vi "read.vi"(7 "timeout (ms)":i32, 8 "error in (no error)":errorcluster, 9 "number of channels":i32, 10 "block size":i32, 11 "FPGAWrapperDL090211Galvo in":refnum<class "FPGAWrapperDL090211Galvo.lvclass">) -> (0 "error out":errorcluster, 1 "channels raw data block":T1, 2 "FIFO full?":bool, 3 "FPGAWrapperDL090211Galvo out":refnum<class "FPGAWrapperDL090211Galvo.lvclass">, 4 "timed out?":bool)   [LabVIEW 2010, in "FPGAWrapperDL090211Galvo.lvclass"]
uses:
  FPGAWrapperDL090211Galvo.lvclass
  common/arrays/pixel_raw_data_array.ctl
  FPGAWrapperDL090211Galvo.lvclass/FPGAWrapperDL090211Galvo.ctl
  <vilib>/rvi/interface/nirviReadWriteControl/nirviReadWriteControl.xnode
  FPGA_VI_ref.ctl
  <vilib>/rvi/interface/common/niFpgaNodeNameForErrorReporting.ctl
  <vilib>/rvi/errors/niLvFpgaWhatHappensToTopLevelVI.ctl
  GenericFPGAWrapper/GenericFPGAWrapper/GenericFPGAWrapper.lvclass
  <vilib>/rvi/interface/nirviMethod/nirviMethod.xnode
  <vilib>/Utility/error.llb/Error Cluster From Error Code.vi
  <vilib>/rvi/errors/niLvFpgaAdjustHostInterfaceError.vi
  NiFpgaLv.dll
panel:
  out "elements remaining in FIFOs":i32[](array[numeric])
  out "FIFO overflow":bool
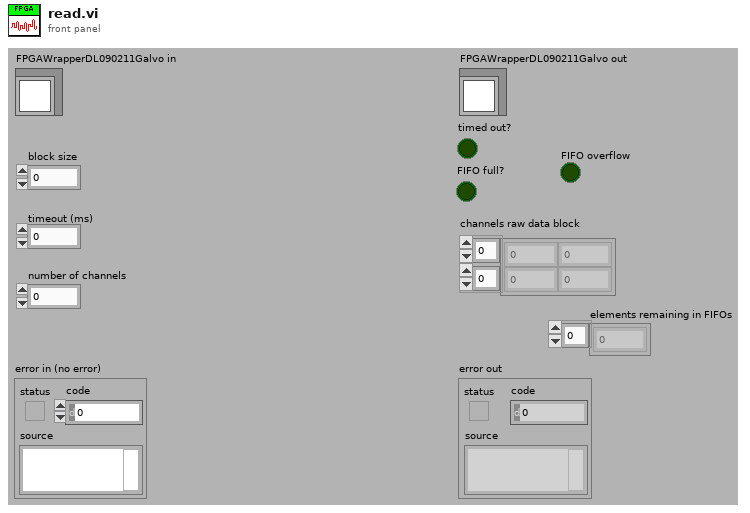
[diagram p1: front panel]
types:
  T1 = typedef "pixel_raw_data_array.ctl" = dbl[][]
  T2 = typedef "niFpgaNodeNameForErrorReporting.ctl" = enum16{"Open FPGA VI Reference", "Read/Write Control", "Invoke Method: Abort", "Invoke Method: Acknowledge IRQ", "Invoke Method: Download", "Invoke Method: FIFO.Configure", "Invoke Method: FIFO.Read", "Invoke Method: FIFO.Start", "Invoke Method: FIFO.Stop", "Invoke Method: FIFO.Write", "Invoke Method: Reset", "Invoke Method: Run", "Invoke Method: Wait on IRQ", "Close FPGA VI Reference"}
  T3 = typedef "niLvFpgaWhatHappensToTopLevelVI.ctl" = enum16{"top level VI scripted behind XNode", "top level VI inlined behind XNode"}
  T4 = typedef "pixel_to_host_enum.ctl" = enum16{"3-channel mode", "4-channel mode"}
  T5 = typedef "FPGAWrapperDL090211Galvo.lvclass/FPGA_VI_ref.ctl" = refnum<k20>
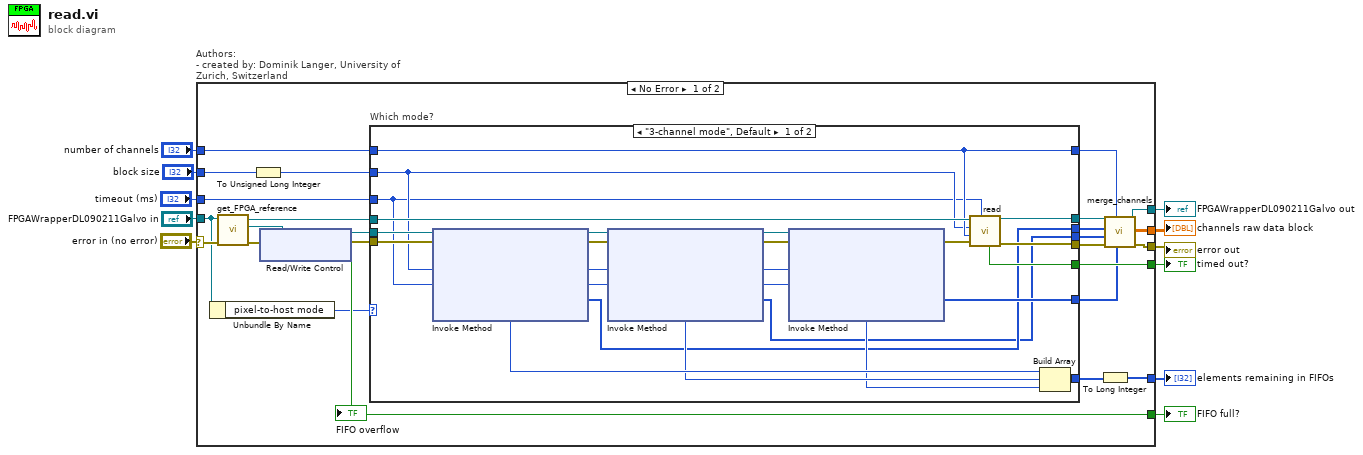
[diagram p0: block diagram]
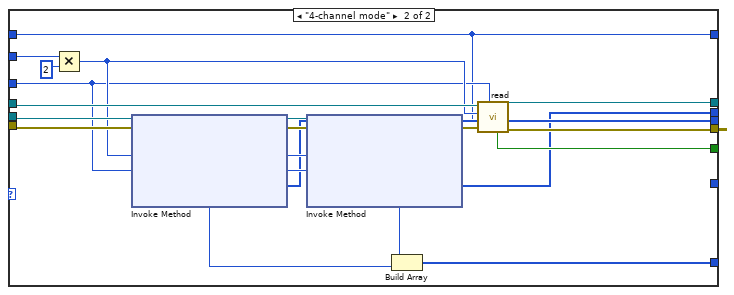
[diagram p2: hidden frame]
diagram:
  n1 = case "Authors: \n- created by: Dominik Langer, University of Zurich, Switzerland" shown="No Error" "error in (no error)" {
    selector: "error in (no error)" -> [w36 w485]
    tunnel: "FPGAWrapperDL090211Galvo in" -> [w13 w486]
    tunnel: "timeout (ms)" -> [w29 _]
    tunnel: "number of channels" -> [w28 _]
    tunnel: "block size" -> [w26 _]
    tunnel: [w30 _] -> w6
    tunnel: [w22 w485] -> w5
    tunnel: [w18 _] -> w4
    tunnel: [w19 w486] -> w3
    tunnel: [w27 _] -> w2
    tunnel: [w23 _] -> w1
    frame No Error {
      n2 = Unbundle By Name(w13) -> ("pixel-to-host mode"=w12:T4)
      n3 = call-dynamic "get_FPGA_reference.vi"("error in (no error)"=w36, "FPGAWrapperDL090211Galvo in"=w13) -> ("error out"=w35:errorcluster, "FPGA VI reference"=w34:T5, "FPGAWrapperDL090211Galvo out"=w31:refnum<class "FPGAWrapperDL090211Galvo.lvclass">)  [unwired: 6 in, 1 out]
      n4 = To Unsigned Long Integer(number=w26) -> (unsigned 32bit integer=w25:u32)
      n5 = xnode "Read/Write Control"("FPGA VI Reference In"=w34, "error in"=w35) -> ("FPGA VI Reference Out"=w33:T5, "error out"=w32:errorcluster, "FIFO overflow"=w27:bool)
      "FIFO overflow" <- w27
      n6 = case "Which mode?" shown="\"3-channel mode\", Default" w12 {
        tunnel: w33 -> [w57 w289]
        tunnel: w32 -> [w56 w290]
        tunnel: w31 -> [w53 w288]
        tunnel: [w43 w282] -> w24
        tunnel: [w52 w285] -> w30
        tunnel: w29 -> [w37 w286]
        tunnel: w28 -> [w40 w277]
        tunnel: [w46 w281] -> w21
        tunnel: [w45 w280] -> w20
        tunnel: w25 -> [w38 w294]
        tunnel: [w39 w279] -> w15
        tunnel: [w41 w278] -> w16
        tunnel: [w42 _] -> w17
        tunnel: [w40 w277] -> w14
        frame "3-channel mode", Default {
          n7 = xnode "Invoke Method"("FPGA VI Reference In"=w57, "error in"=w56, "Number of Elements"=w38, "Timeout (ms)"=w37) -> ("FPGA VI Reference Out"=w54:T5, "error out"=w55:errorcluster, "Data"=w41:u16[], "Elements Remaining"=w48:u32)
          n8 = xnode "Invoke Method"("FPGA VI Reference In"=w54, "error in"=w55, "Number of Elements"=w38, "Timeout (ms)"=w37) -> ("FPGA VI Reference Out"=w51:T5, "error out"=w50:errorcluster, "Data"=w39:u16[], "Elements Remaining"=w47:u32)
          n9 = xnode "Invoke Method"("FPGA VI Reference In"=w51, "error in"=w50, "Number of Elements"=w38, "Timeout (ms)"=w37) -> ("error out"=w49:errorcluster, "Data"=w42:u16[], "Elements Remaining"=w44:u32)  [unwired: 1 out]
          n10 = call-parent "read.vi"("timeout (ms)"=w37, "error in (no error)"=w49, "number of channels"=w40, "block size"=w38, "GenericFPGAWrapper in"=w53) -> ("error out"=w46:errorcluster, "GenericFPGAWrapper out"=w45:refnum<class "FPGAWrapperDL090211Galvo.lvclass">, "timed out?"=w52:bool)  [unwired: 2 in, 2 out]
          n11 = Build Array(w48, w47, w44) -> (w43:u32[])
        }
        frame "4-channel mode" {
          n12 = Multiply(x=w294, y=u32 2 ("x")) -> (x*y=w287:u32)
          n13 = xnode "Invoke Method"("FPGA VI Reference In"=w289, "error in"=w290, "Number of Elements"=w287, "Timeout (ms)"=w286) -> ("FPGA VI Reference Out"=w291:T5, "error out"=w292:errorcluster, "Data"=w279:u16[], "Elements Remaining"=w283:u32)
          n14 = xnode "Invoke Method"("FPGA VI Reference In"=w291, "error in"=w292, "Number of Elements"=w287, "Timeout (ms)"=w286) -> ("error out"=w293:errorcluster, "Data"=w278:u16[], "Elements Remaining"=w284:u32)  [unwired: 1 out]
          n15 = Build Array(w284, w283) -> (w282:u32[])
          n16 = call-parent "read.vi"("timeout (ms)"=w286, "error in (no error)"=w293, "number of channels"=w277, "block size"=w287, "GenericFPGAWrapper in"=w288) -> ("error out"=w281:errorcluster, "GenericFPGAWrapper out"=w280:refnum<class "FPGAWrapperDL090211Galvo.lvclass">, "timed out?"=w285:bool)  [unwired: 2 in, 2 out]
        }
      }
      n17 = To Long Integer(number=w24) -> (32bit integer=w23:i32[])
      n18 = call-dynamic "merge_channels.vi"("FIFO_3"=w17, "number of channels"=w14, "error in (no error)"=w21, "FIFO_2"=w15, "FIFO_1"=w16, "DL090211FPGAWrapper in"=w20) -> ("error out"=w22:errorcluster, "channels raw data block"=w18:T1, "DL090211FPGAWrapper out"=w19:refnum<class "FPGAWrapperDL090211Galvo.lvclass">)  [unwired: 3 in]
    }
    frame Error {
    }
  }
  "error out" <- w5
  "FPGAWrapperDL090211Galvo out" <- w3
  "FIFO full?" <- w2
  "channels raw data block" <- w4
  "timed out?" <- w6
  "elements remaining in FIFOs" <- w1
